vi "Notifiy Counter.vi"(9 "Blackboard Group":string="A", 10 "Time (ms)":u32=20, 11 "Blackboard in":refnum<class "Blackboard.lvclass">) -> (2 "Value":refnum<class "Abs_I32 Integer.lvclass">[](array[class]), 3 "Node Out":refnum<class "bt_Node.lvclass">)   [LabVIEW 2021]
uses:
  Source/BT.lvlib
  Source/Support/Nodes/Decorators/Repeater/Support/Finish On - Type.ctl
  Source/Support/Nodes/Decorators/Repeater/bt_Repeater.lvclass
  Source/Blackboard/Blackboard.lvclass
  Source/Blackboard/Get Value Type/Get I32.vi
  <vilib>/TSA/Abstract Data Classes/Functions/Math/Support/Increment/I32/Method.vi
  <vilib>/TSA/Abstract Data Classes/Functions/Math/Support/Increment/I32/Increment_I32.lvclass
  <vilib>/TSA/Abstract Data Classes/Constants/Support/I32/I32.vi
  <vilib>/TSA/Abstract Data Classes/Constants/Support/I32/Const_I32.lvclass
  <vilib>/TSA/Abstract Data Classes/Functions/Compare/Support/Greater Equal/I32/Method.vi
  <vilib>/TSA/Abstract Data Classes/Functions/Compare/Support/Greater Equal/I32/Greater Equal_I32.lvclass
  <vilib>/TSA/Abstract Data Classes/Abs_Types/I32 Integer/Abs_I32 Integer.lvclass
  C:/Program Files (x86)/National Instruments/LabVIEW 2021/vi.lib/TSA/Abstract Data Classes/Abs_Types/Integer/Abs_Integer.lvclass
  C:/Program Files (x86)/National Instruments/LabVIEW 2021/vi.lib/TSA/Abstract Data Classes/Abs_Types/Numeric/Abs_Numeric.lvclass
  C:/Program Files (x86)/National Instruments/LabVIEW 2021/vi.lib/TSA/Abstract Data Classes/Abs_Types/Value/Abs_Value.lvclass
  C:/Program Files (x86)/National Instruments/LabVIEW 2021/vi.lib/TSA/Abstract Data Classes/Abs_Types/Type/Abs_Type.lvclass
  C:/Program Files (x86)/National Instruments/LabVIEW 2021/vi.lib/TSA/Abstract Data Classes/Abs_Types/I32 Integer/Abs_I32 Integer.lvclass
  Source/Support/Nodes/abs_Node/bt_Node.lvclass
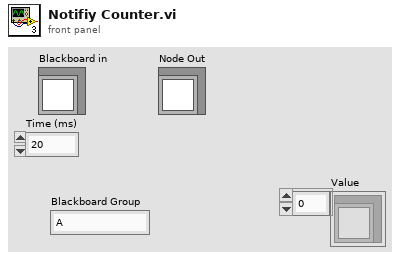
[diagram p1: front panel]
types:
  T1 = typedef "BT.lvlib/bt_Repeater.lvclass/Finish On - Type.ctl" = enum16{"Success", "Failure", "Never"}
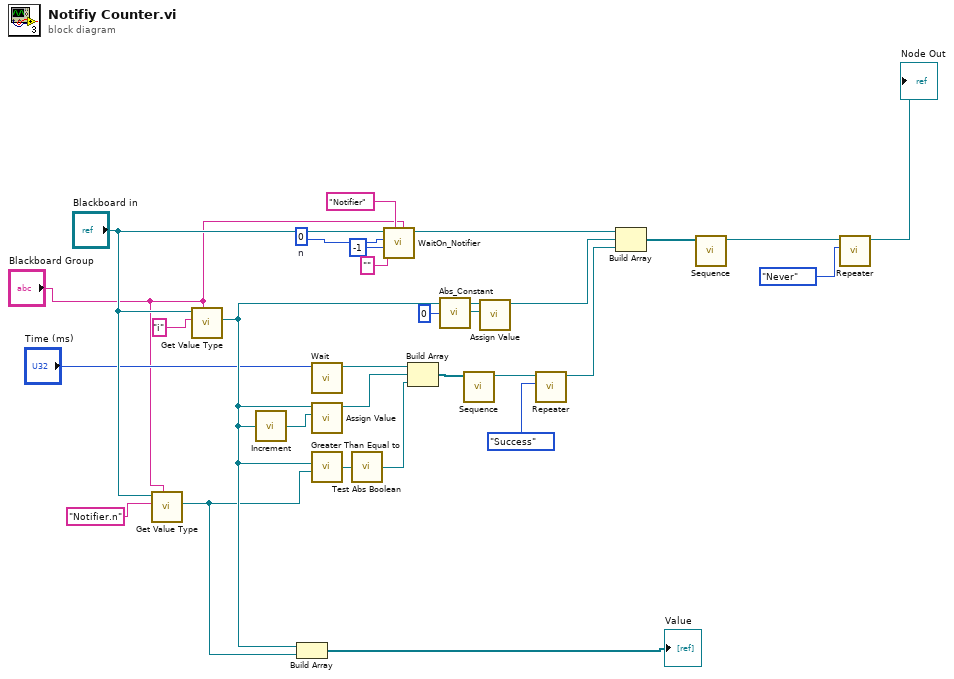
[diagram p0: block diagram]
diagram:
  w27 = 0  # n
  n1 = call-poly "Get Value Type.vi"("Tag Group"="Blackboard Group", "Tag"="Notifier.n", "Blackboard in"="Blackboard in") -> ("Value"=w3:refnum<class "Abs_I32 Integer.lvclass">)  [unwired: 5 in, 3 out]
  n2 = call-poly "Get Value Type.vi"("Tag Group"="Blackboard Group", "Tag"="i", "Blackboard in"="Blackboard in") -> ("Value"=w22:refnum<class "Abs_I32 Integer.lvclass">)  [unwired: 5 in, 3 out]
  n3 = call-poly <vilib>:"Increment.vi"("Value"=w22) -> ("Result"=w17:refnum<class "Abs_I32 Integer.lvclass">)  [unwired: 4 in]
  n4 = Build Array(w22, w3) -> (→"Value":refnum<class "Abs_I32 Integer.lvclass">[])
  n5 = call "Wait.vi"("Time (ms)"="Time (ms)") -> ("Node Out"=w23:refnum<class "bt_Node.lvclass">)  [unwired: 10 in]
  n6 = call "Assign Value.vi"("Assigned Value"=w17, "Value"=w22) -> ("Node Out"=w18:refnum<class "bt_Node.lvclass">)  [unwired: 9 in]
  n7 = call-poly <vilib>:"Greater Than Equal to.vi"("Value B"=w3, "Value A"=w22) -> ("Result"=w19:refnum<class "Abs_Boolean.lvclass">)  [unwired: 4 in]
  n8 = call "Test Abs Boolean.vi"("Abs_Boolean.lvclass"=w19) -> ("abs_Node"=w20:refnum<class "bt_Node.lvclass">)  [unwired: 4 in]
  n9 = call "WaitOn_Notifier.vi"("Blackboard Group"="Blackboard Group", "Notifier Name"="Notifier" ("Name"), "Tag Root"="", "Timeout (ms)"=-1, "Message Type"=w27, "bt_Blackboard in"="Blackboard in") -> ("Node Out"=w28:refnum<class "bt_Node.lvclass">)  [unwired: 4 in, 1 out]
  n10 = Build Array(w23, w18, w20) -> (w12:refnum<class "bt_Node.lvclass">[])
  n11 = call-poly <vilib>:"Abs_Constant.vi"("Value"=0 ("n")) -> ("Constant"=w16:refnum<class "Abs_I32 Integer.lvclass">)  [unwired: 4 in]
  n12 = call "Sequence.vi"("Nodes"=w12) -> ("Node"=w11:refnum<class "bt_Node.lvclass">)  [unwired: 10 in]
  n13 = call "Assign Value.vi"("Assigned Value"=w16, "Value"=w22) -> ("Node Out"=w21:refnum<class "bt_Node.lvclass">)  [unwired: 9 in]
  n14 = call "Repeater.vi"("Finish On"=Finish_On_-_Type."Success", "Node In"=w11) -> ("Node Out"=w10:refnum<class "bt_Node.lvclass">)  [unwired: 9 in]
  n15 = Build Array(w28, w21, w10) -> (w8:refnum<class "bt_Node.lvclass">[])
  n16 = call "Sequence.vi"("Nodes"=w8) -> ("Node"=w9:refnum<class "bt_Node.lvclass">)  [unwired: 10 in]
  n17 = call "Repeater.vi"("Finish On"=Finish_On_-_Type."Never", "Node In"=w9) -> ("Node Out"=→"Node Out":refnum<class "bt_Node.lvclass">)  [unwired: 9 in]
